vi "is Transmission Ended.vi"(8 "error in (no error)":errorcluster, 10 "Board":u16, 11 "identifier":string) -> (0 "error out":errorcluster, 3 "function return":u32)   [LabVIEW 2015, in "XGL_DPP.lvlib"]
doc: "EXTERN DECLSPEC uint32_t CALL_CONV isTransmissionEnded(const char * identifier, uint16_t Board);"
uses:
  XGL_DPP.lvlib
  XGL_DPP.dll
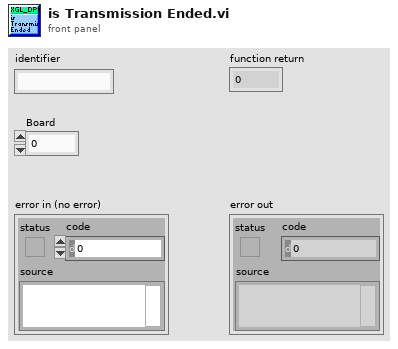
[diagram p1: front panel]
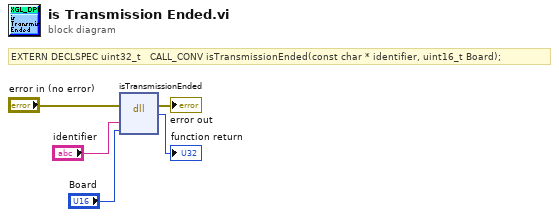
[diagram p0: block diagram]
diagram:
  # "EXTERN DECLSPEC uint32_t   CALL_CONV isTransmissionEnded(const char * identifier, uint16_t Board);"
  n1 = dll-call lib="D:/Users/XRF/Desktop/Scanning Software_Demokritos_2015_v7/libs/Vis_2/XGL_DPP.*" fn="isTransmissionEnded"(error in="error in (no error)", "identifier"="identifier", "Board"="Board") -> (error out=→"error out":errorcluster, →"function return":u32)  [unwired: 4 in, 1 out]
